vi "stack_remove.vi"(8 "error in (no error)":errorcluster, 10 "index":i32, 11 "Lua in":refnum<class "Lua.lvclass">) -> (0 "error out":errorcluster, 3 "Lua out":refnum<class "Lua.lvclass">)   [LabVIEW 2020, in "Lua for LabVIEW.lvlib" / "Lua.lvclass"]
doc: "Accepts any acceptable index, or 0, and sets the stack top to this index. If the new top is larger than the old one, then the new elements are filled with nil. If index is 0, then all stack elements are removed."
uses:
  Lua.lvclass
  Lua.lvclass/Lua.ctl
  lib/lua.dll/lua.dll.lvlib
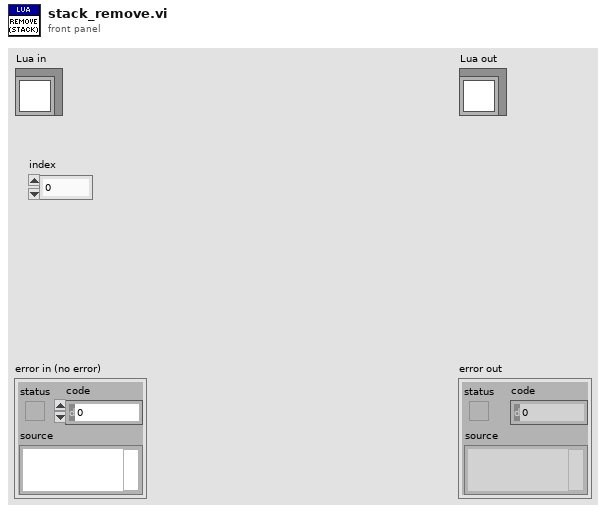
[diagram p1: front panel]
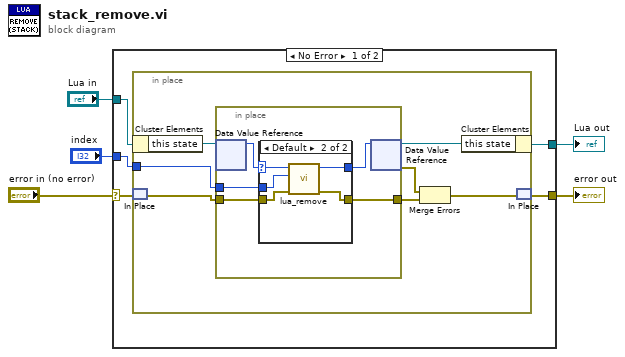
[diagram p0: block diagram]
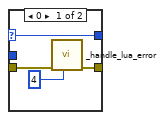
[diagram p2: hidden frame]
diagram:
  n1 = case shown="No Error" "error in (no error)" {
    selector: "error in (no error)" -> [w7 w33]
    tunnel: [w8 w33] -> w4
    tunnel: [w9 w32] -> w2
    tunnel: "Lua in" -> [w10 w32]
    tunnel: "index" -> [w6 _]
    frame No Error {
      n2 = in-place {
        in-place-border: w6 -> [w16]
        n3 = in-place-cluster #1(w10) -> ("this state"=w15:refnum<data-value>)
        n4 = in-place-match #2(w7) -> (w17:errorcluster)
        n5 = in-place {
          in-place-border: w17 -> [w22]
          in-place-border: [w21] -> w13
          in-place-border: w16 -> [w20]
          n6 = in-place-dvr #3(w15) -> (w19:u64)  [unwired: 1 out]
          n7 = case shown="Default" w19 {
            selector: w19 -> [w26 w30]
            tunnel: [w26 w31] -> w18
            tunnel: w22 -> [w23 w29]
            tunnel: [w24 w28] -> w21
            tunnel: w20 -> [_ w27]
            frame 0 {
              n8 = call "_handle_lua_error.vi"("lua status"=4 ("lua_load errcode"), "error in (no error)"=w23) -> ("error out"=w24:errorcluster)  [unwired: 9 in]
            }
            frame Default {
              n9 = call "lua_remove.vi"("error in (no error)"=w29, "index"=w27, "lua_state_p"=w30) -> ("error out"=w28:errorcluster, "lua_state_p out"=w31:u64)  [unwired: 7 in]
            }
          }
          n10 = in-place-dvr #3(w18) -> (w11:refnum<data-value>, w14:errorcluster)
        }
        n11 = Merge Errors(w14, w13) -> (w12:errorcluster)
        n12 = in-place-cluster #1("this state"=w11) -> (w9:refnum<class "Lua.lvclass">)
        n13 = in-place-match #2(w12) -> (w8:errorcluster)
      }
    }
    frame Error {
    }
  }
  "error out" <- w4
  "Lua out" <- w2
